vi "LUCS001RT_GPS_Decoder_GPRMB.vi"(8 "error in (no error)":errorcluster, 9 "SerialData:$GPRMB":string=",A,0.01,L,OriginWP,AVALON,3320.800,N,11819.360,W,033.7,247.2,234,A*06", 11 "GPS DataIn":T1={"WayPointDataGood"=TRUE, "Waypoint:XTE"=0.01, "Waypoint:SteeringDirection"="L", "WayPoint:OriginID"="", "Waypoint:DestinationID"="", "DestinationWaypoint.Latitude.Deg"=0, "DestinationWaypoint.Latitude.Min"=0.0, "DestinationWaypointLatitude.North/South"="", "DestinationWaypointLongitude.Deg"=0, "DestinationWaypointLongitude.Min"=0.0, "DestinationWaypointLongitude.East/West"="", "RangeToDestination(NauticalMiles)"=0.0, "TrueBearingToDestination"=33.7, "VelocityTowardsDestination(Knots)"=0.0, "ArrivalAlarm"=TRUE, "ITOW"=247, "TAcc"=0, "LON"=0.0, "LAT"=0.0, "HEIGHT"=0, "HMSL"=0, "Hacc"=0, "Vacc"=0, "MSTOW"=0, "FixType"=0, "ECEF_X_Coor"=0, "ECEF_Y_Coor"=0, "ECEF_Z_Coor"=0, "Pacc"=0, "ECEF_X_Vlsty"=0, "ECEF_Y_Vlsty"=0, "ECEF_Z_Vlsty"=0, "Sacc"=0, "PosDOP"=0, "#SatsInNavSol"=0, "NED_NVsty"=0, "NED_Evsty"=0, "NED_DNvsty"=0, "Speed(3-D)"=0, "GSpeed(2-D)"=0, "Heading(2-D)"=0.0, "CAcc"=0, "Nano"=0, "Year"=0, "Month"=0, "Day"=0, "Hour"=0, "Min"=0, "Sec"=0, "UTC Valid"=0} {"UTC Valid" items=["UTC not valid", "Valid Time of Week", "Valid Week Number", "NA", "Valid UTC"]; "CAcc" format="%.0f°"; "Heading(2-D)" format="%0.6f°"; "GSpeed(2-D)" format="%.0f cm/s"; "Speed(3-D)" format="%.0f cm/s"; "NED_DNvsty" format="%.0f cm/s"; "NED_Evsty" format="%.0f cm/s"; "NED_NVsty" format="%.0f cm/s"; "Sacc" format="%.0f cm/s"; "ECEF_Z_Vlsty" format="%.0f cm/s"; "ECEF_Y_Vlsty" format="%.0f cm/s"; "ECEF_X_Vlsty" format="%.0f cm/s"; "FixType" items=["No Fix", "Dead Reckoning Only", "2D-Fix", "3D-Fix", "GPS + Dead Reckoning", "Time Only Fix", "RESERVED"]; "Vacc" format="%.0f mm"; "Hacc" format="%.0f mm"; "HMSL" format="%d mm"; "HEIGHT" format="%.0f mm"; "LAT" format="%#.6f"; "LON" format="%#.6f"; "Waypoint:XTE" format="%#.2f"}) -> (0 "error out":errorcluster, 3 "GPS DataOut":T1={"WayPointDataGood"=TRUE, "Waypoint:XTE"=0.01, "Waypoint:SteeringDirection"="L", "WayPoint:OriginID"="", "Waypoint:DestinationID"="", "DestinationWaypoint.Latitude.Deg"=0, "DestinationWaypoint.Latitude.Min"=0.0, "DestinationWaypointLatitude.North/South"="", "DestinationWaypointLongitude.Deg"=0, "DestinationWaypointLongitude.Min"=0.0, "DestinationWaypointLongitude.East/West"="", "RangeToDestination(NauticalMiles)"=0.0, "TrueBearingToDestination"=33.7, "VelocityTowardsDestination(Knots)"=0.0, "ArrivalAlarm"=TRUE, "ITOW"=247, "TAcc"=0, "LON"=0.0, "LAT"=0.0, "HEIGHT"=0, "HMSL"=0, "Hacc"=0, "Vacc"=0, "MSTOW"=0, "FixType"=0, "ECEF_X_Coor"=0, "ECEF_Y_Coor"=0, "ECEF_Z_Coor"=0, "Pacc"=0, "ECEF_X_Vlsty"=0, "ECEF_Y_Vlsty"=0, "ECEF_Z_Vlsty"=0, "Sacc"=0, "PosDOP"=0, "#SatsInNavSol"=0, "NED_NVsty"=0, "NED_Evsty"=0, "NED_DNvsty"=0, "Speed(3-D)"=0, "GSpeed(2-D)"=0, "Heading(2-D)"=0.0, "CAcc"=0, "Nano"=0, "Year"=0, "Month"=0, "Day"=0, "Hour"=0, "Min"=0, "Sec"=0, "UTC Valid"=0} {"UTC Valid" items=["UTC not valid", "Valid Time of Week", "Valid Week Number", "NA", "Valid UTC"]; "CAcc" format="%.0f°"; "Heading(2-D)" format="%0.6f°"; "GSpeed(2-D)" format="%.0f cm/s"; "Speed(3-D)" format="%.0f cm/s"; "NED_DNvsty" format="%.0f cm/s"; "NED_Evsty" format="%.0f cm/s"; "NED_NVsty" format="%.0f cm/s"; "Sacc" format="%.0f cm/s"; "ECEF_Z_Vlsty" format="%.0f cm/s"; "ECEF_Y_Vlsty" format="%.0f cm/s"; "ECEF_X_Vlsty" format="%.0f cm/s"; "FixType" items=["No Fix", "Dead Reckoning Only", "2D-Fix", "3D-Fix", "GPS + Dead Reckoning", "Time Only Fix", "RESERVED"]; "Vacc" format="%.0f mm"; "Hacc" format="%.0f mm"; "HMSL" format="%d mm"; "HEIGHT" format="%.0f mm"; "LAT" format="%#.6f"; "LON" format="%#.6f"; "Waypoint:XTE" format="%#.2f"})   [LabVIEW 2020]
uses:
  LUCS001RT_GPS_Data.ctl
panel:
  # "WAYPOINT"
  # "CURRENT POSITION"
  # "WAYPOINT"
  # "CURRENT POSITION"
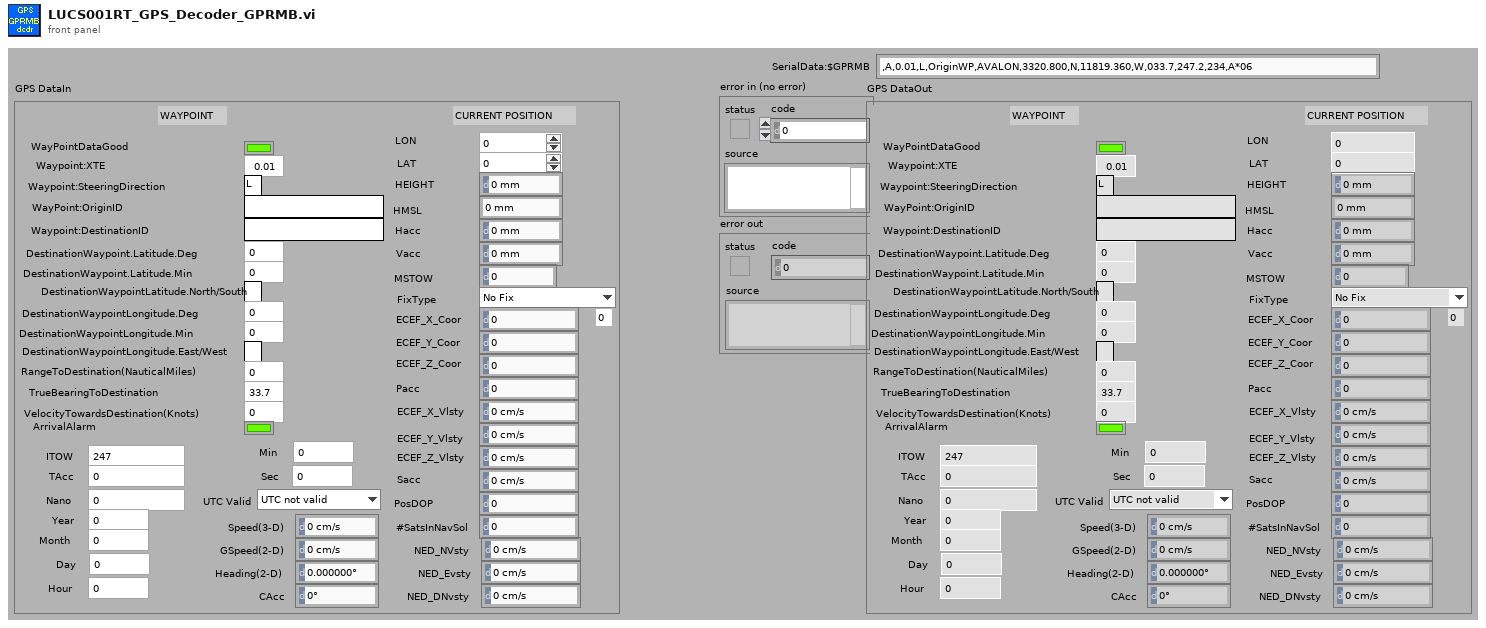
[diagram p1: front panel]
types:
  T1 = typedef "LUCS001RT_GPS_Data.ctl" = cluster{"WayPointDataGood":bool, "Waypoint:XTE":dbl, "Waypoint:SteeringDirection":string, "WayPoint:OriginID":string, "Waypoint:DestinationID":string, "DestinationWaypoint.Latitude.Deg":i32, "DestinationWaypoint.Latitude.Min":dbl, "DestinationWaypointLatitude.North/South":string, "DestinationWaypointLongitude.Deg":i32, "DestinationWaypointLongitude.Min":dbl, "DestinationWaypointLongitude.East/West":string, "RangeToDestination(NauticalMiles)":dbl, "TrueBearingToDestination":dbl, "VelocityTowardsDestination(Knots)":dbl, "ArrivalAlarm":bool, "ITOW":u32, "TAcc":u32, "LON":dbl, "LAT":dbl, "HEIGHT":i32, "HMSL":i32, "Hacc":u32, "Vacc":u32, "MSTOW":u32, "FixType":u8, "ECEF_X_Coor":i32, "ECEF_Y_Coor":i32, "ECEF_Z_Coor":i32, "Pacc":u32, "ECEF_X_Vlsty":i32, "ECEF_Y_Vlsty":i32, "ECEF_Z_Vlsty":i32, "Sacc":u32, "PosDOP":u16, "#SatsInNavSol":u8, "NED_NVsty":i32, "NED_Evsty":i32, "NED_DNvsty":i32, "Speed(3-D)":u32, "GSpeed(2-D)":u32, "Heading(2-D)":dbl, "CAcc":u32, "Nano":i32, "Year":u16, "Month":u8, "Day":u8, "Hour":u8, "Min":u8, "Sec":u8, "UTC Valid":u8}
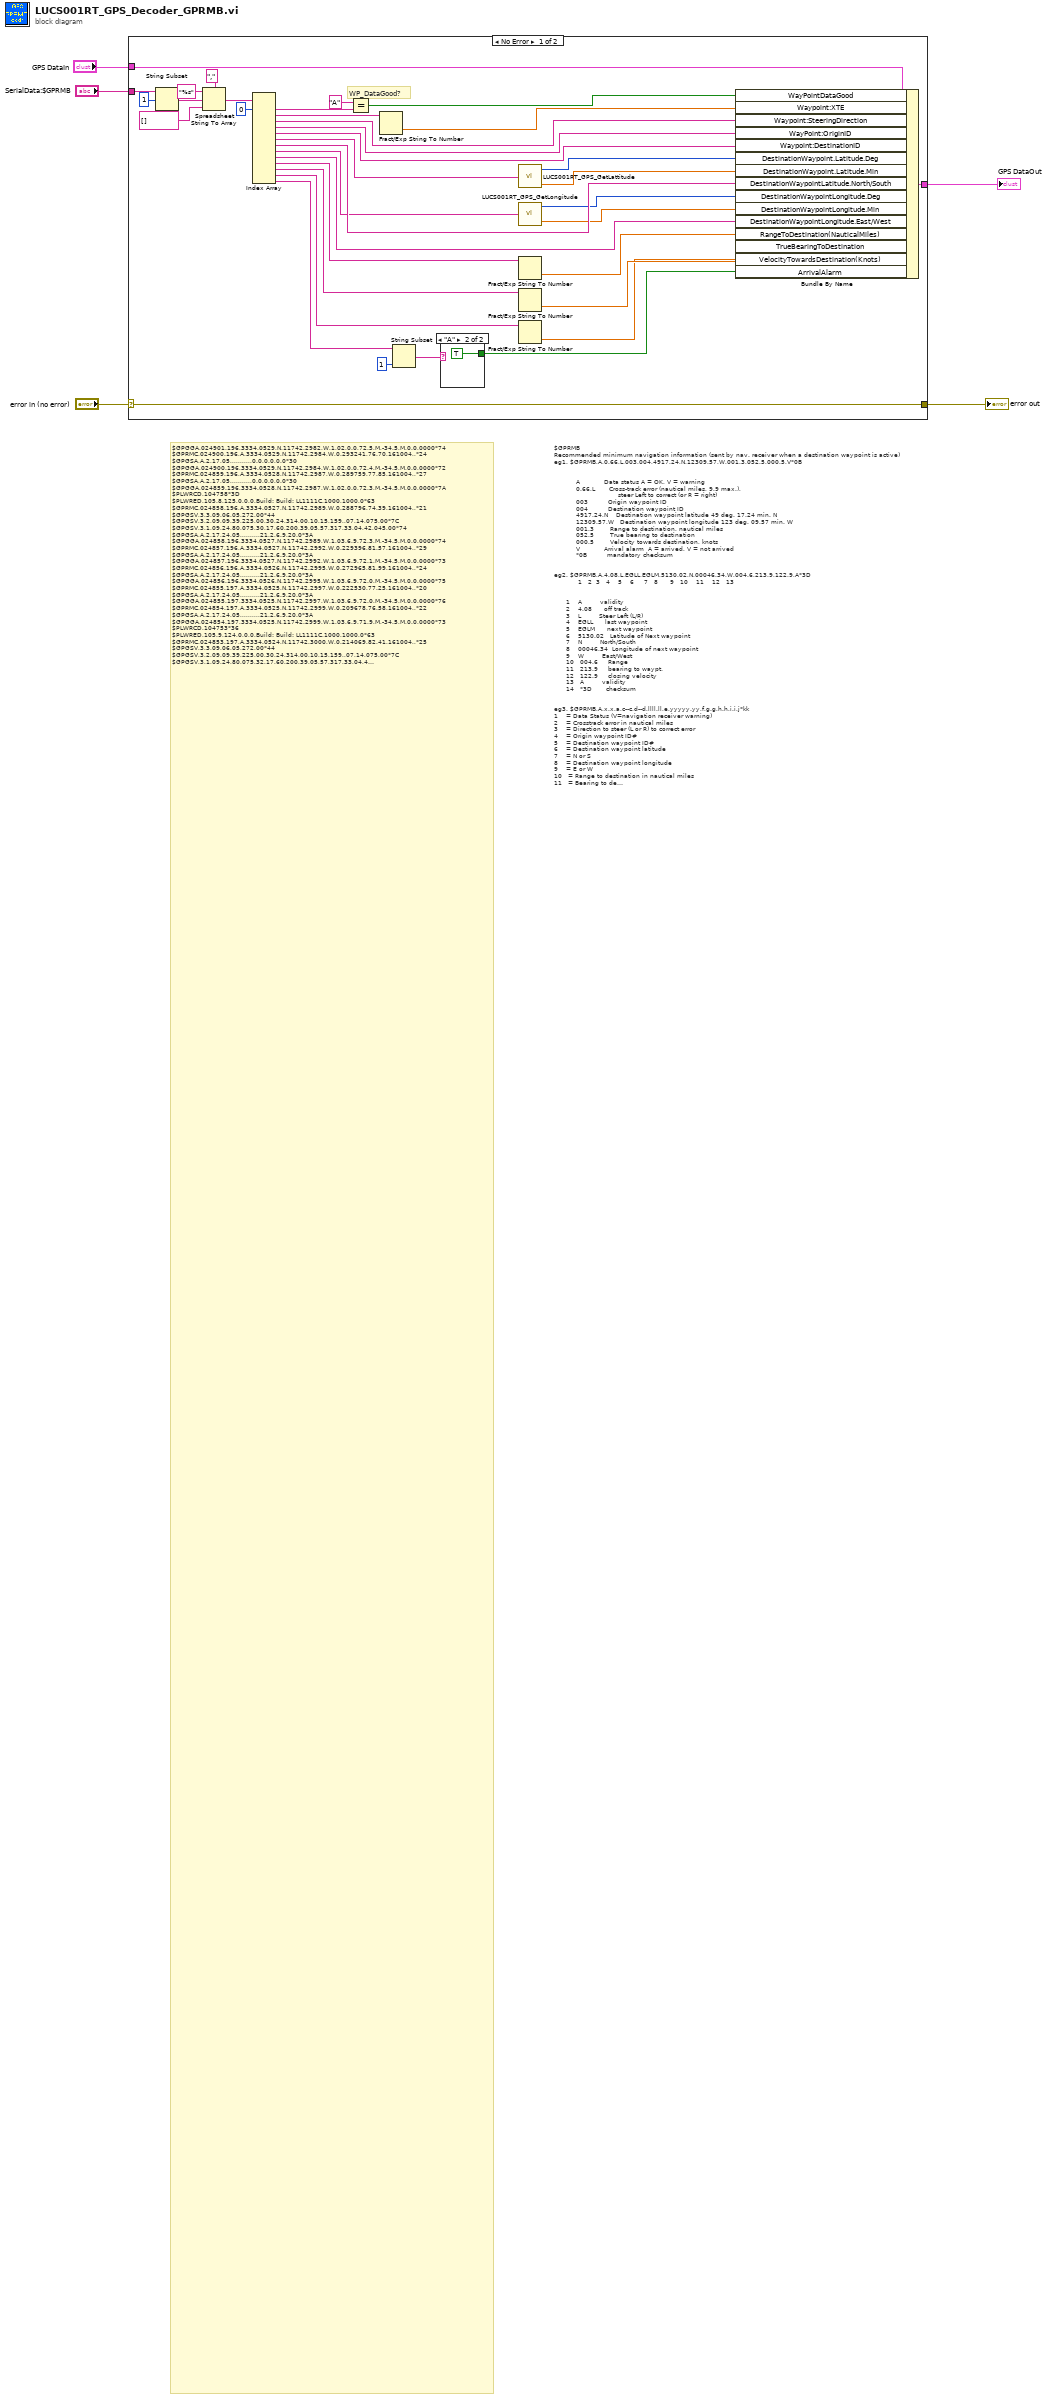
[diagram p0: block diagram]
diagram:
  # "$GPGGA,024901.196,3334.0529,N,11742.2982,W,1,02,0.0,72.5,M,-34.5,M,0.0,0000*74\n$GPRMC,024900.196,A,3334.0529,N,11742.2984,W,0.293241,76.70,161004,,*24\n$GPGSA,A,2,17,05,,,,,,,,,,,0.0,0.0,0.0*30\n$GPGGA,024900.196,3334.0529,N,11742.2984,W,1,02,0.0,72.4,M,-34.5,M,0.0,0000*72\n$GPRMC,024859.196,A,3334.0528,N,11742.2987,W,0.289759,77.85,161004,,*27\n$GPGSA,A,2,17,05,,,,,,,,,,,0.0,0.0,0.0*30\n$GPGGA,024859.196,3334.0528,N,11742.2987,W,1,02,0.0,72.3,M,-34.5,M,0.0,0000*7A\n$PLWRCD,104758*3D\n$PLWRED,105.8,125,0,0,0,Build: Build: LL1111C,1000,1000,0*63\n$GPRMC,024858.196,A,3334.0527,N,11742.2989,W,0.288796,74.39,161004,,*21\n$GPGSV,3,3,09,06,05,272,00*44\n$GPGSV,3,2,09,09,39,225,00,30,24,314,00,10,15,159,,07,14,075,00*7C\n$GPGSV,3,1,09,24,80,075,30,17,60,200,39,05,57,317,33,04,42,045,00*74\n$GPGSA,A,2,17,24,05,,,,,,,,,,21.2,6.9,20.0*3A\n$GPGGA,024858.196,3334.0527,N,11742.2989,W,1,03,6.9,72.3,M,-34.5,M,0.0,0000*74\n$GPRMC,024857.196,A,3334.0527,N,11742.2992,W,0.229396,81.57,161004,,*29\n$GPGSA,A,2,17,24,05,,,,,,,,,,21.2,6.9,20.0*3A\n$GPGGA,024857.196,3334.0527,N,11742.2992,W,1,03,6.9,72.1,M,-34.5,M,0.0,0000*73\n$GPRMC,024856.196,A,3334.0526,N,11742.2995,W,0.272965,81.99,161004,,*24\n$GPGSA,A,2,17,24,05,,,,,,,,,,21.2,6.9,20.0*3A\n$GPGGA,024856.196,3334.0526,N,11742.2995,W,1,03,6.9,72.0,M,-34.5,M,0.0,0000*75\n$GPRMC,024855.197,A,3334.0525,N,11742.2997,W,0.222530,77.25,161004,,*20\n$GPGSA,A,2,17,24,05,,,,,,,,,,21.2,6.9,20.0*3A\n$GPGGA,024855.197,3334.0525,N,11742.2997,W,1,03,6.9,72.0,M,-34.5,M,0.0,0000*76\n$GPRMC,024854.197,A,3334.0525,N,11742.2999,W,0.209678,76.58,161004,,*22\n$GPGSA,A,2,17,24,05,,,,,,,,,,21.2,6.9,20.0*3A\n$GPGGA,024854.197,3334.0525,N,11742.2999,W,1,03,6.9,71.9,M,-34.5,M,0.0,0000*73\n$PLWRCD,104753*36\n$PLWRED,105.9,124,0,0,0,Build: Build: LL1111C,1000,1000,0*63\n$GPRMC,024853.197,A,3334.0524,N,11742.3000,W,0.214069,82.41,161004,,*25\n$GPGSV,3,3,09,06,05,272,00*44\n$GPGSV,3,2,09,09,39,225,00,30,24,314,00,10,15,159,,07,14,075,00*7C\n$GPGSV,3,1,09,24,80,075,32,17,60,200,39,05,57,317,33,04,42,045,21*75\n$GPGSA,A,2,17,24,05,,,,,,,,,,21.2,6.9,20.0*3A\n$GPGGA,024853.197,3334.0524,N,11742.3000,W,1,03,6.9,71.8,M,-34.5,M,0.0,0000*7C\n$GPRMC,024852.197,A,3334.0524,N,11742.3001,W,0.122901,61.77,161004,,*2C\n$GPGSA,A,2,17,24,05,,,,,,,,,,21.2,6.9,20.0*3A\n$GPGGA,024852.197,3334.0524,N,11742.3001,W,1,03,6.9,71.8,M,-34.5,M,0.0,0000*7C\n$GPRMC,024851.197,A,3334.0523,N,11742.3001,W,0.120608,69.73,161004,,*20\n$GPGSA,A,2,17,24,05,,,,,,,,,,21.2,7.0,20.0*32\n$GPGGA,024851.197,3334.0523,N,11742.3001,W,1,03,7.0,71.8,M,-34.5,M,0.0,0000*70\n$GPRMC,024850.197,A,3334.0523,N,11742.3001,W,0.169479,83.95,161004,,*24\n$GPGSA,A,2,17,24,05,,,,,,,,,,21.2,7.0,20.0*32\n$GPGGA,024850.197,3334.0523,N,11742.3001,W,1,03,7.0,71.9,M,-34.5,M,0.0,0000*70\n$GPRMC,024849.197,A,3334.0523,N,11742.3002,W,0.201276,72.87,161004,,*26\n$GPGSA,A,2,17,24,05,,,,,,,,,,21.2,7.0,20.0*32\n$GPGGA,024849.197,3334.0523,N,11742.3002,W,1,03,7.0,71.9,M,-34.5,M,0.0,0000*7B\n$PLWRCD,104749*3D\n$PLWRED,105.9,124,0,0,0,Build: Build: LL1111C,1000,1000,0*63\n$GPRMC,024848.197,A,3334.0523,N,11742.3003,W,0.157569,80.86,161004,,*23\n$GPGSV,3,3,09,06,05,272,00*44\n$GPGSV,3,2,09,09,39,225,23,30,24,314,00,10,15,159,,07,14,075,00*7D\n$GPGSV,3,1,09,24,80,075,32,17,60,200,38,05,57,317,33,04,42,045,21*74\n$GPGSA,A,2,17,24,05,,,,,,,,,,21.2,7.0,20.0*32\n$GPGGA,024848.197,3334.0523,N,11742.3003,W,1,03,7.0,71.8,M,-34.5,M,0.0,0000*7A\n$GPRMC,024847.197,A,3334.0523,N,11742.3003,W,0.132289,89.85,161004,,*2C\n$GPGSA,A,2,17,24,05,,,,,,,,,,21.2,7.0,20.0*32\n$GPGGA,024847.197,3334.0523,N,11742.3003,W,1,03,7.0,71.8,M,-34.5,M,0.0,0000*75\n$GPRMC,024846.197,A,3334.0523,N,11742.3004,W,0.167397,82.13,161004,,*20\n$GPGSA,A,2,17,24,05,,,,,,,,,,21.2,7.0,20.0*32\n$GPGGA,024846.197,3334.0523,N,11742.3004,W,1,03,7.0,71.8,M,-34.5,M,0.0,0000*73\n$GPRMC,024845.197,A,3334.0523,N,11742.3004,W,0.144840,89.69,161004,,*25\n$GPGSA,A,2,17,24,05,,,,,,,,,,21.2,7.0,20.0*32\n$GPGGA,024845.197,3334.0523,N,11742.3004,W,1,03,7.0,71.8,M,-34.5,M,0.0,0000*70\n$GPRMC,024844.197,A,3334.0522,N,11742.3004,W,0.102003,58.93,161004,,*21\n$GPGSA,A,2,17,24,05,,,,,,,,,,21.2,7.0,20.0*32\n$GPGGA,024844.197,3334.0522,N,11742.3004,W,1,03,7.0,71.8,M,-34.5,M,0.0,0000*70\n$PLWRCD,104745*31\n$PLWRED,105.9,124,0,0,0,Build: Build: LL1111C,1000,1000,0*63\n$GPRMC,024843.197,A,3334.0522,N,11742.3005,W,0.156643,73.79,161004,,*29\n$GPGSV,3,3,09,06,05,272,00*44\n$GPGSV,3,2,09,09,39,225,23,30,24,314,00,10,14,159,,07,14,075,00*7C\n$GPGSV,3,1,09,24,80,077,33,17,59,200,38,05,57,317,32,04,42,045,27*7A\n$GPGSA,A,2,17,24,05,,,,,,,,,,21.2,7.0,20.0*32\n$GPGGA,024843.197,3334.0522,N,11742.3005,W,1,03,7.0,71.7,M,-34.5,M,0.0,0000*79\n$GPRMC,024842.197,A,3334.0522,N,11742.3005,W,0.142581,75.26,161004,,*2C\n$GPGSA,A,2,17,24,05,,,,,,,,,,21.2,7.0,20.0*32\n$GPGGA,024842.197,3334.0522,N,11742.3005,W,1,03,7.0,71.7,M,-34.5,M,0.0,0000*78\n$GPRMC,024841.197,A,3334.0522,N,11742.3006,W,0.148497,77.15,161004,,*22\n$GPGSA,A,2,17,24,05,,,,,,,,,,21.2,7.0,20.0*32\n$GPGGA,024841.197,3334.0522,N,11742.3006,W,1,03,7.0,71.6,M,-34.5,M,0.0,0000*79\n$GPRMC,024840.198,A,3334.0523,N,11742.3007,W,0.176740,83.59,161004,,*2B\n$GPGSA,A,2,17,24,05,,,,,,,,,,21.2,7.0,20.0*32\n$GPGGA,024840.198,3334.0523,N,11742.3007,W,1,03,7.0,71.5,M,-34.5,M,0.0,0000*74\n$GPRMC,024839.198,A,3334.0523,N,11742.3008,W,0.161318,78.50,161004,,*28\n$GPGSA,A,2,17,24,05,,,,,,,,,,21.2,7.0,20.0*32\n$GPGGA,024839.198,3334.0523,N,11742.3008,W,1,03,7.0,71.3,M,-34.5,M,0.0,0000*73\n$PLWRCD,104741*35\n$PLWRED,105.9,124,0,0,0,Build: Build: LL1111C,1000,1000,0*63\n$GPRMC,024838.198,A,3334.0523,N,11742.3009,W,0.123798,83.07,161004,,*24\n$GPGSV,3,3,09,06,05,272,00*44\n$GPGSV,3,2,09,09,39,225,25,30,24,314,00,10,14,159,,07,14,075,00*7A\n$GPGSV,3,1,09,24,80,077,32,17,59,200,38,05,57,317,31,04,42,045,27*78\n$GPGSA,A,2,17,24,05,,,,,,,,,,21.2,7.0,20.0*32\n$GPGGA,024838.198,3334.0523,N,11742.3009,W,1,03,7.0,71.1,M,-34.5,M,0.0,0000*71\n$GPRMC,024837.198,A,3334.0523,N,11742.3009,W,0.130354,74.06,161004,,*24\n$GPGSA,A,3,17,04,24,05,,,,,,,,,6.1,2.3,5.6*36\n$GPGGA,024837.198,3334.0523,N,11742.3009,W,1,04,2.3,70.9,M,-34.5,M,0.0,0000*76\n$GPRMC,024836.198,A,3334.0524,N,11742.3006,W,0.094691,61.44,161004,,*2C\n$GPGSA,A,3,17,04,24,05,,,,,,,,,6.1,2.3,5.6*36\n$GPGGA,024836.198,3334.0524,N,11742.3006,W,1,04,2.3,69.8,M,-34.5,M,0.0,0000*76\n$GPRMC,024835.198,A,3334.0524,N,11742.2998,W,0.148941,81.19,161004,,*24\n$GPGSA,A,3,17,04,24,05,,,,,,,,,6.1,2.3,5.6*36\n$GPGGA,024835.198,3334.0524,N,11742.2998,W,1,04,2.3,68.0,M,-34.5,M,0.0,0000*73\n$GPRMC,024834.198,A,3334.0524,N,11742.2991,W,0.163408,64.25,161004,,*21\n$GPGSA,A,2,17,24,05,,,,,,,,,,21.2,7.0,20.0*32\n$GPGGA,024834.198,3334.0524,N,11742.2991,W,1,03,7.0,66.8,M,-34.5,M,0.0,0000*7C\n$PLWRCD,104736*35\n$PLWRED,106.0,124,0,0,0,Build: Build: LL1111C,1000,1000,0*69\n$GPRMC,024833.198,A,3334.0523,N,11742.2991,W,0.108364,51.82,161004,,*2A\n$GPGSV,3,3,09,06,05,272,00*44\n$GPGSV,3,2,09,09,39,225,00,30,24,314,00,10,14,159,,07,14,075,00*7D\n$GPGSV,3,1,09,24,80,077,33,17,59,200,37,05,57,317,30,04,42,045,00*72\n$GPGSA,A,2,17,24,05,,,,,,,,,,21.2,7.0,20.0*32\n$GPGGA,024833.198,3334.0523,N,11742.2991,W,1,03,7.0,66.9,M,-34.5,M,0.0,0000*7D\n$GPRMC,024832.198,A,3334.0523,N,11742.2990,W,0.159191,81.42,161004,,*27\n$GPGSA,A,2,17,24,05,,,,,,,,,,21.2,7.0,20.0*32\n$GPGGA,024832.198,3334.0523,N,11742.2990,W,1,03,7.0,67.0,M,-34.5,M,0.0,0000*75\n$GPRMC,024831.198,A,3334.0523,N,11742.2989,W,0.131473,75.66,161004,,*26\n$GPGSA,A,2,17,24,05,,,,,,,,,,21.2,7.0,20.0*32\n$GPGGA,024831.198,3334.0523,N,11742.2989,W,1,03,7.0,67.1,M,-34.5,M,0.0,0000*7F\n$GPRMC,024830.198,A,3334.0522,N,11742.2989,W,0.105221,78.44,161004,,*2D\n$GPGSA,A,2,17,24,05,,,,,,,,,,21.2,7.0,20.0*32\n$GPGGA,024830.198,3334.0522,N,11742.2989,W,1,03,7.0,67.2,M,-34.5,M,0.0,0000*7C\n$GPRMC,024829.198,A,3334.0522,N,11742.2988,W,0.118962,65.72,161004,,*2D\n$GPGSA,A,2,17,24,05,,,,,,,,,,21.2,7.0,20.0*32\n$GPGGA,024829.198,3334.0522,N,11742.2988,W,1,03,7.0,67.4,M,-34.5,M,0.0,0000*73\n$PLWRCD,104731*32\n$PLWRED,106.0,124,0,0,0,Build: Build: LL1111C,1000,1000,0*69\n$GPRMC,024828.198,A,3334.0521,N,11742.2987,W,0.078376,47.32,161004,,*2C\n$GPGSV,3,3,09,06,05,272,00*44\n$GPGSV,3,2,09,09,39,225,00,30,24,314,00,10,14,159,,07,14,075,00*7D\n$GPGSV,3,1,09,24,80,077,33,17,59,200,36,05,57,317,31,04,42,045,27*77\n$GPGSA,A,2,17,24,05,,,,,,,,,,21.2,7.0,20.0*32\n$GPGGA,024828.198,3334.0521,N,11742.2987,W,1,03,7.0,67.5,M,-34.5,M,0.0,0000*7F\n$GPRMC,024827.198,A,3334.0521,N,11742.2987,W,0.138951,75.88,161004,,*29\n$GPGSA,A,2,17,24,05,,,,,,,,,,21.2,7.0,20.0*32\n$GPGGA,024827.198,3334.0521,N,11742.2987,W,1,03,7.0,67.5,M,-34.5,M,0.0,0000*70\n$GPRMC,024826.198,A,3334.0521,N,11742.2987,W,0.127507,75.06,161004,,*2F\n$GPGSA,A,2,17,24,05,,,,,,,,,,21.2,7.0,20.0*32\n$GPGGA,024826.198,3334.0521,N,11742.2987,W,1,03,7.0,67.5,M,-34.5,M,0.0,0000*71\n$GPRMC,024825.199,A,3334.0521,N,11742.2988,W,0.120407,73.18,161004,,*2D\n$GPGSA,A,2,17,24,05,,,,,,,,,,21.2,7.0,20.0*32\n$GPGGA,024825.199,3334.0521,N,11742.2988,W,1,03,7.0,67.5,M,-34.5,M,0.0,0000*7C\n$GPRMC,024824.199,A,3334.0521,N,11742.2988,W,0.144431,91.14,161004,,*2B\n$GPGSA,A,2,17,24,05,,,,,,,,,,21.2,7.0,20.0*32\n$GPGGA,024824.199,3334.0521,N,11742.2988,W,1,03,7.0,67.5,M,-34.5,M,0.0,0000*7D\n$PLWRCD,104727*35\n$PLWRED,106.0,124,0,0,0,Build: Build: LL1111C,1000,1000,0*69\n$GPRMC,024823.199,A,3334.0521,N,11742.2989,W,0.081524,94.61,161004,,*27\n$GPGSV,3,3,09,06,05,272,00*44\n$GPGSV,3,2,09,09,39,225,25,30,24,314,00,10,14,159,,07,14,075,00*7A\n$GPGSV,3,1,09,24,80,077,34,17,59,200,35,05,57,317,31,04,42,045,27*73\n$GPGSA,A,2,17,24,05,,,,,,,,,,21.2,7.1,20.0*33\n$GPGGA,024823.199,3334.0521,N,11742.2989,W,1,03,7.1,67.5,M,-34.5,M,0.0,0000*7A\n$GPRMC,024822.199,A,3334.0521,N,11742.2989,W,0.118461,82.09,161004,,*2E\n$GPGSA,A,3,17,04,24,05,,,,,,,,,6.1,2.3,5.6*36\n$GPGGA,024822.199,3334.0521,N,11742.2989,W,1,04,2.3,67.5,M,-34.5,M,0.0,0000*7B\n$GPRMC,024821.199,A,3334.0522,N,11742.2989,W,0.118978,80.44,161004,,*20\n$GPGSA,A,2,17,24,05,,,,,,,,,,21.2,7.1,20.0*33\n$GPGGA,024821.199,3334.0522,N,11742.2989,W,1,03,7.1,67.7,M,-34.5,M,0.0,0000*79\n$GPRMC,024820.199,A,3334.0523,N,11742.2989,W,0.170025,80.46,161004,,*2D\n$GPGSA,A,3,17,04,24,05,,,,,,,,,6.1,2.3,5.6*36\n$GPGGA,024820.199,3334.0523,N,11742.2989,W,1,04,2.3,67.6,M,-34.5,M,0.0,0000*78\n$GPRMC,024819.199,A,3334.0522,N,11742.2990,W,0.124653,47.89,161004,,*20\n$GPGSA,A,3,17,04,24,05,,,,,,,,,6.1,2.3,5.6*36\n$GPGGA,024819.199,3334.0522,N,11742.2990,W,1,04,2.3,66.7,M,-34.5,M,0.0,0000*7B\n$PLWRCD,104723*31\n$PLWRED,250.0,124,0,0,0,Build: Build: LL1111C,1000,1000,0*69\n$GPRMC,024818.199,A,3334.0521,N,11742.2985,W,0.301036,88.94,161004,,*29\n$GPGSV,3,3,09,06,05,272,00*44\n$GPGSV,3,2,09,09,39,225,25,30,24,314,00,10,14,159,,07,14,075,00*7A\n$GPGSV,3,1,09,24,80,077,29,17,59,200,33,05,57,317,27,04,42,045,28*71\nVÖ\n†xx†¦"
  # "$GPRMB\nRecommended minimum navigation information (sent by nav. receiver when a destination waypoint is active) \neg1. $GPRMB,A,0.66,L,003,004,4917.24,N,12309.57,W,001.3,052.5,000.5,V*0B\n\n\n           A            Data status A = OK, V = warning\n           0.66,L       Cross-track error (nautical miles, 9.9 max.),\n                                steer Left to correct (or R = right)\n           003          Origin waypoint ID\n           004          Destination waypoint ID\n           4917.24,N    Destination waypoint latitude 49 deg. 17.24 min. N\n           12309.57,W   Destination waypoint longitude 123 deg. 09.57 min. W\n           001.3        Range to destination, nautical miles\n           052.5        True bearing to destination\n           000.5        Velocity towards destination, knots\n           V            Arrival alarm  A = arrived, V = not arrived\n           *0B          mandatory checksum\n\n\neg2. $GPRMB,A,4.08,L,EGLL,EGLM,5130.02,N,00046.34,W,004.6,213.9,122.9,A*3D\n            1   2  3   4    5    6     7   8      9   10    11    12   13\n\n  \n      1    A         validity\n      2    4.08      off track\n      3    L         Steer Left (L/R)\n      4    EGLL      last waypoint\n      5    EGLM      next waypoint\n      6    5130.02   Latitude of Next waypoint\n      7    N         North/South\n      8    00046.34  Longitude of next waypoint\n      9    W         East/West\n      10   004.6     Range\n      11   213.9     bearing to waypt.\n      12   122.9     closing velocity\n      13   A         validity\n      14   *3D       checksum\n\n\neg3. $GPRMB,A,x.x,a,c--c,d--d,llll.ll,e,yyyyy.yy,f,g.g,h.h,i.i,j*kk\n1    = Data Status (V=navigation receiver warning)\n2    = Crosstrack error in nautical miles\n3    = Direction to steer (L or R) to correct error\n4    = Origin waypoint ID#\n5    = Destination waypoint ID#\n6    = Destination waypoint latitude\n7    = N or S\n8    = Destination waypoint longitude\n9    = E or W\n10   = Range to destination in nautical miles\n11   = Bearing to destination, degrees True\n12   = Destination closing velocity in knots\n13   = Arrival status; (A=entered or perpendicular passed)\n14   = Checksum"
  n1 = case shown="No Error" "error in (no error)" {
    selector: "error in (no error)" -> [w32 w44]
    tunnel: "SerialData:$GPRMB" -> [w33 _]
    tunnel: [w32 w44] -> w3
    tunnel: [w23 _] -> w2
    tunnel: "GPS DataIn" -> [w12 _]
    frame No Error {
      # "WP_DataGood?"
      n2 = String Subset(string=w33, offset (0)=1) -> (substring=w35:string)  [unwired: 1 in]
      n3 = Spreadsheet String To Array(delimiter (Tab)=",", format string="%s", spreadsheet string=w35, array type (2D Dbl)=string[] []) -> (array=w39:string[])
      n4 = Index Array(array=w39, index #1=0 ("index")) -> (element #1=w40:string, element #2=w42:string, element #3=w21:string, element #4=w20:string, element #5=w19:string, element #6=w11:string, element #7=w18:string, element #8=w8:string, element #9=w17:string, element #10=w30:string, element #11=w29:string, element #12=w28:string, element #13=w26:string)  [unwired: 12 in]
      n5 = Equal?(x="A", y=w40) -> (x = y?=w24:bool)
      n6 = Fract/Exp String To Number(string=w42) -> (number=w22:dbl)  [unwired: 3 in, 1 out]
      n7 = String Subset(string=w26, length (rest)=1 ("length (rest)")) -> (substring=w25:string)  [unwired: 1 in]
      n8 = case shown="\"A\"" w25 {
        tunnel: [_ TRUE] -> w13
        frame "V", Default {
        }
        frame "A" {
        }
      }
      n9 = call "LUCS001RT_GPS_GetLattitude.vi"("LattitudeString"=w11) -> ("Lattitude.Degrees"=w10:i32, "Lattitude.Minutes"=w9:dbl)  [unwired: 5 in]
      n10 = call "LUCS001RT_GPS_GetLongitude.vi"("LongitudeString"=w8) -> ("Longitude.Degrees"=w7:i32, "Longitude.Minutes"=w6:dbl)  [unwired: 5 in]
      n11 = Fract/Exp String To Number(string=w30) -> (number=w16:dbl)  [unwired: 3 in, 1 out]
      n12 = Fract/Exp String To Number(string=w29) -> (number=w15:dbl)  [unwired: 3 in, 1 out]
      n13 = Fract/Exp String To Number(string=w28) -> (number=w14:dbl)  [unwired: 3 in, 1 out]
      n14 = Bundle By Name(cluster=w12, "WayPointDataGood"=w24, "Waypoint:XTE"=w22, "Waypoint:SteeringDirection"=w21, "WayPoint:OriginID"=w20, "Waypoint:DestinationID"=w19, "DestinationWaypoint.Latitude.Deg"=w10, "DestinationWaypoint.Latitude.Min"=w9, "DestinationWaypointLatitude.North/South"=w18, "DestinationWaypointLongitude.Deg"=w7, "DestinationWaypointLongitude.Min"=w6, "DestinationWaypointLongitude.East/West"=w17, "RangeToDestination(NauticalMiles)"=w16, "TrueBearingToDestination"=w15, "VelocityTowardsDestination(Knots)"=w14, "ArrivalAlarm"=w13) -> (w23:T1)
    }
    frame Error {
    }
  }
  "error out" <- w3
  "GPS DataOut" <- w2
